vi "UpdateUserInterface.vi"(8 "error in (no error)":errorcluster, 10 "DataExchange":T1, 11 "Controller Template in":refnum<class "Controller Template.lvclass">) -> (0 "error out":errorcluster, 2 "DataExchange Out":T1, 3 "Controller Template out":refnum<class "Controller Template.lvclass">)   [LabVIEW 2020, in "Controller Template.lvlib" / "Controller Template.lvclass"]
uses:
  Controller Template.lvclass
  Model/Hardware Abstraction Layer/Component/Device/Device/DataExchange.ctl
  Controller Template.lvclass/Controller Template.ctl
  Model/Hardware Abstraction Layer/Component/GenericActor/GenericActor/GenericController.lvclass
  Interface/DataListener/DataListener.lvclass
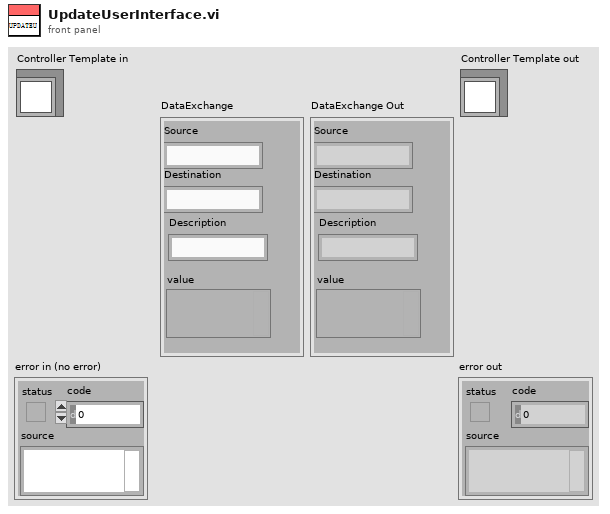
[diagram p1: front panel]
types:
  T1 = typedef "DataListener.lvclass/DataExchange.ctl" = cluster{"Source":string, "Destination":string, "Description":string, "value":variant}
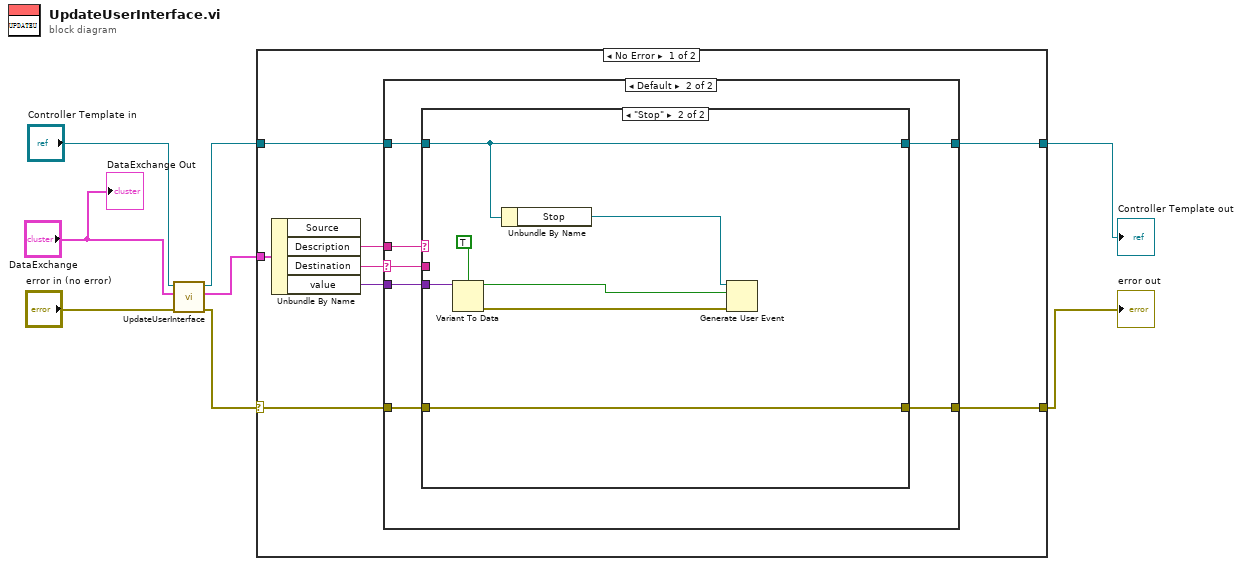
[diagram p0: block diagram]
diagram:
  n1 = call-parent "UpdateUserInterface.vi"("error in (no error)"="error in (no error)", "DataExchange"="DataExchange", "GenericController in"="Controller Template in") -> ("error out"=w7:errorcluster, "DataExchange Out"=w1:T1, "GenericController out"=w2:refnum<class "Controller Template.lvclass">)  [unwired: 6 in]
  n2 = case shown="No Error" w7 {
    selector: w7 -> [w11 w36]
    tunnel: [w10 w36] -> w4
    tunnel: [w12 w35] -> w3
    tunnel: w2 -> [w13 w35]
    tunnel: w1 -> [w16 _]
    frame No Error {
      n3 = Unbundle By Name(w16) -> ("Description"=w14:string, "Destination"=w9:string, "value"=w15:variant)  [unwired: 1 out]
      n4 = case shown="Default" w9 {
        selector: w9 -> [_ w19]
        tunnel: w15 -> [_ w25]
        tunnel: w14 -> [_ w24]
        tunnel: w13 -> [w18 w23]
        tunnel: [w18 w22] -> w12
        tunnel: w11 -> [w17 w21]
        tunnel: [w17 w20] -> w10
        frame "duplicate this case" {
        }
        frame Default {
          n5 = case shown="\"Stop\"" w24 {
            tunnel: w25 -> [_ w34]
            tunnel: [w27 w29] -> w22
            tunnel: w23 -> [w27 w29]
            tunnel: [w26 w28] -> w20
            tunnel: w21 -> [w26 w28]
            tunnel: w19 -> [_ _]
            frame Default {
            }
            frame "Stop" {
              n6 = Variant To Data(type=TRUE, Variant=w34) -> (data=w32:bool, error out=w30:errorcluster)  [unwired: 1 in]
              n7 = Unbundle By Name(w29) -> ("Stop"=w33:refnum<user-event>)
              n8 = Generate User Event(user event=w33, event data cluster=w32, error in=w30) -> ()  [unwired: 1 in, 2 out]
            }
          }
        }
      }
    }
    frame Error {
    }
  }
  "error out" <- w4
  "Controller Template out" <- w3
  "DataExchange Out" <- "DataExchange"
